vi "Tidy Up MCLB UI.vi"(8 "error in (no error)":errorcluster, 10 "Event Log":refnum<vi>, 11 "VI in":refnum<vi>) -> (0 "error out":errorcluster)   [LabVIEW 2020, in "Event Manager.lvlib"]
doc: "____\nHAMPEL SOFTWARE ENGINEERING v2.6.0 (2023-12-19 10:54)"
uses:
  Event Manager.lvlib
  Libraries/hse-libraries/Source/hse-ui/hse-ui.lvlib
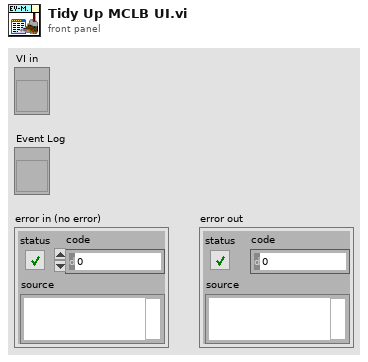
[diagram p1: front panel]
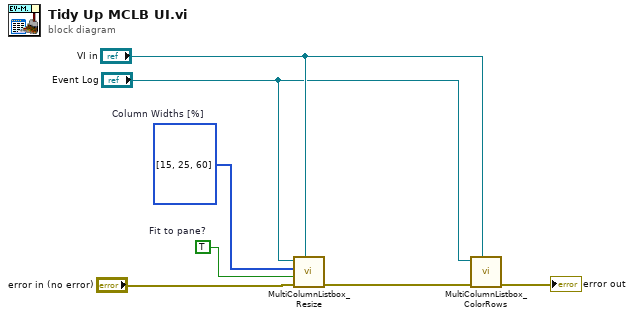
[diagram p0: block diagram]
diagram:
  w2 = u32[] [15, 25, 60]  # Column Widths [%]
  w1 = TRUE  # Fit to pane?
  n1 = call "MultiColumnListbox_Resize.vi"("Parent VI Reference"="VI in", "error in (no error)"="error in (no error)", "Fit to pane?"=w1, "Column Widths [%]"=w2, "MCListbox Refnum"="Event Log") -> ("error out"=w6:errorcluster)  [unwired: 6 in]
  n2 = call "MultiColumnListbox_ColorRows.vi"("Parent VI Reference"="VI in", "error in"=w6, "MCListbox Refnum"="Event Log") -> ("error out"=→"error out":errorcluster)  [unwired: 8 in]
